vi "Write_Control_Values.vi"(8 "error in (no error)":errorcluster, 10 "Path of VI with Controls to change":path, 11 "Control Value:Get All 2":cluster{"Name":string, "Variant Data":variant}[](array[cluster])) -> (0 "error out":errorcluster)   [LabVIEW 2013]
doc: "Illustrates how to read a configuration settings file. Run Write Configuration (INI) File.vi. Then run this VI."
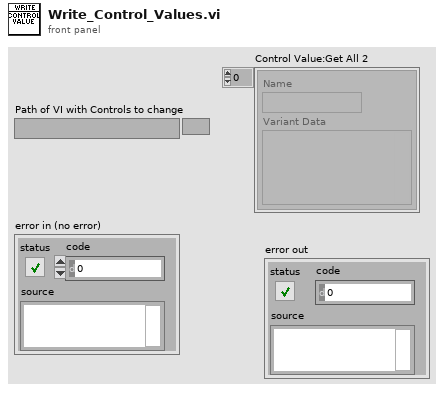
[diagram p1: front panel]
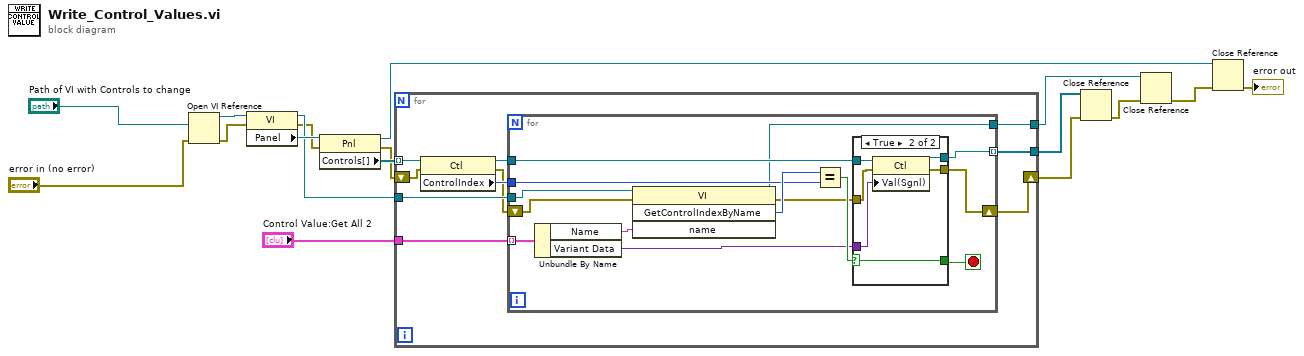
[diagram p0: block diagram]
diagram:
  n1 = Open VI Reference(vi path="Path of VI with Controls to change", error in (no error)="error in (no error)") -> (vi reference=w12:refnum<vi>, error out=w4:errorcluster)  [unwired: 4 in]
  n2 = property class="VI"(reference=w12, error in=w4) -> (reference out=w10:refnum<vi>, error out=w7:errorcluster, "Panel"=w15:refnum<vi>)
  n3 = property class="Pnl"(reference=w15, error in=w7) -> (reference out=w9:refnum<vi>, error out=w8:errorcluster, "Controls[]"=w16:refnum<vi>[])
  n4 = for {
    tunnel: "Control Value:Get All 2" -> [w27]
    tunnel: w16 -> [w26] mode=indexing
    tunnel: [w23] -> w13
    tunnel: w10 -> [w22]
    tunnel: [w21] -> w11
    shift-right: [w20] -> w3
    shift-left: w8 -> [w18]
    n5 = property class="Ctl"(reference=w26, error in=w18) -> (reference out=w24:refnum<vi>, error out=w19:errorcluster, "ControlIndex"=w25:i32)
    n6 = for {
      tunnel: w27 -> [w40] mode=indexing
      tunnel: w25 -> [w38]
      tunnel: w24 -> [w34]
      tunnel: [w33] -> w23 mode=indexing
      tunnel: w22 -> [w32]
      tunnel: [w31] -> w21
      shift-right: [w30] -> w20
      shift-left: w19 -> [w28]
      stop <- w36 stop-if-true
      n7 = Unbundle By Name(w40) -> ("Name"=w41:string, "Variant Data"=w35:variant)
      n8 = invoke class="VI" method="GetControlIndexByName"(reference=w32, error in=w28, "name"=w41) -> (reference out=w31:refnum<vi>, error out=w29:errorcluster, "GetControlIndexByName"=w39:i32)  [unwired: 1 in, 1 out]
      n9 = Equal?(x=w39, y=w38) -> (x = y?=w37:bool)
      n10 = case shown="True" w37 {
        selector: w37 -> [w44 w50]
        tunnel: [w44 w50] -> w36
        tunnel: w35 -> [_ w49]
        tunnel: w34 -> [w43 w48]
        tunnel: [w43 w47] -> w33
        tunnel: [w42 w46] -> w30
        tunnel: w29 -> [w42 w45]
        frame False {
        }
        frame True {
          n11 = property class="Ctl"(reference=w48, error in=w45, "Val(Sgnl)"=w49) -> (reference out=w47:refnum<vi>, error out=w46:errorcluster)
        }
      }
    }
  }
  n12 = Close Reference(reference=w13, error in (no error)=w3) -> (error out=w2:errorcluster)
  n13 = Close Reference(reference=w11, error in (no error)=w2) -> (error out=w1:errorcluster)
  n14 = Close Reference(reference=w9, error in (no error)=w1) -> (error out=→"error out":errorcluster)
